vi "Create.vi"   [LabVIEW 2018, in "Toolkit.lvlib" / "Agent.lvclass"]
doc: "Creates a new Agent object. This allocates memory that must be explicitly deallocated, or freed, later in the application using the Destroy VI."
uses:
  Agent.lvclass
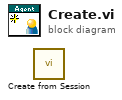
[diagram p0: block diagram]
diagram:
  n1 = call "Create from Session.vi"() -> ()  [unwired: 10 in, 2 out]
